vi "FringeScanner.vi"() -> ()   [LabVIEW 2009, in "FringeScanner.lvlib"]
uses:
  FringeScanner.lvlib
  Nicmos/Controls/NICMOS.READOUT.ctl
panel:
  in  "Wavelength":dbl[unit]=1.3e-06
  in  "Frame per fringe":dbl=5.0
  in  "STOP button":bool
  in  "UPDATE button":bool
  out "OPD per pixel":dbl[unit]
  out "Actual":T1
  in  "Autcollimation":bool=TRUE
  out "OPD stroke":dbl[unit]
  in  "Requested":T1={"Readout"=100, "Deglitch"=10, "Framerate"=200.0, "Bank"=2}
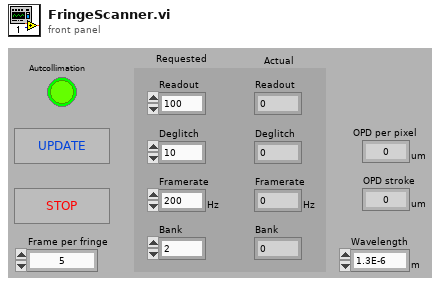
[diagram p1: front panel]
types:
  T1 = typedef "NICMOS.READOUT.ctl" = cluster{"Readout":i32, "Deglitch":i32, "Framerate":dbl[unit], "Bank":i32}
  T2 = typedef "PIEZO.WAVE.ctl" = cluster{"Speed":dbl[unit], "Stiffness (0.95)":dbl, "Linear Stroke":dbl[unit], "Delay":dbl[unit]}
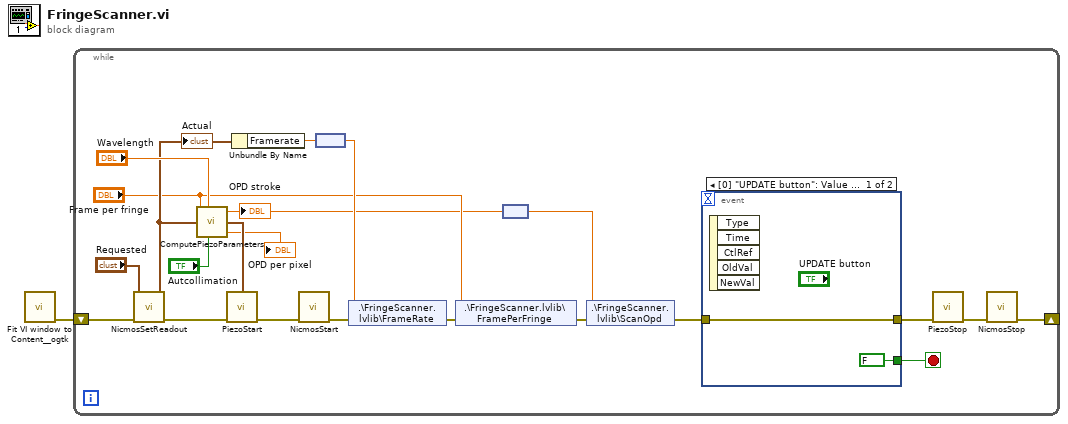
[diagram p0: block diagram]
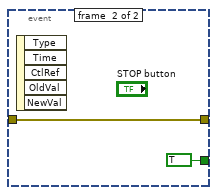
[diagram p2: hidden frame]
diagram:
  n1 = call <userlib>:"Fit VI window to Content__ogtk.vi"() -> ("error out"=w1:errorcluster)  [unwired: 6 in, 1 out]
  n2 = while {
    shift-right: [w22] -> _
    shift-left: w1 -> [w23]
    stop <- w12 stop-if-true
    n3 = call "NicmosSetReadout.vi"("READOUT in"="Requested", "error in (no error)"=w23) -> ("READOUT out"=w11:T1, "error out"=w18:errorcluster)  [unwired: 6 in]
    "Actual" <- w11
    n4 = call "ComputePiezoParameters.vi"("Frame per fringe"="Frame per fringe", "Wavelength"="Wavelength", "READOUT"=w11, "Autcollimation"="Autcollimation") -> ("OPD stroke"=w3:dbl[unit], "WAVE"=w16:T2, "OPD per pixel"=→"OPD per pixel":dbl[unit])  [unwired: 1 in]
    "OPD stroke" <- w3
    n5 = call "PiezoStart.vi"("WAVE"=w16, "error in (no error)"=w18) -> ("error out"=w17:errorcluster)  [unwired: 7 in]
    n6 = Unbundle By Name(w11) -> ("Framerate"=w10:dbl[unit])
    n7 = call "NicmosStart.vi"("error in (no error)"=w17) -> ("error out"=w9:errorcluster)  [unwired: 8 in]
    n8 = node(w10) -> (w8:dbl)
    n9 = shared-variable ".\\FringeScanner.lvlib\\FrameRate"(w8, error in=w9) -> (error out=w7:errorcluster)
    n10 = shared-variable ".\\FringeScanner.lvlib\\FramePerFringe"("Frame per fringe", error in=w7) -> (error out=w6:errorcluster)
    n11 = node(w3) -> (w2:dbl)
    n12 = shared-variable ".\\FringeScanner.lvlib\\ScanOpd"(w2, error in=w6) -> (error out=w5:errorcluster)
    n13 = event shown="[0] \"UPDATE button\": Value Change" {
      selector: _ -> [_ _]
      dyn-events: _ -> [_ _]
      timeout: _ -> [_ _]
      tunnel: w5 -> [w25 w27]
      tunnel: [w25 w27] -> w13
      tunnel: [FALSE TRUE] -> w12
      event #0 {
        n14 = event-data() -> ()  [unwired: 1 in, 5 out]
      }
      event #1 {
        n15 = event-data() -> ()  [unwired: 1 in, 5 out]
      }
    }
    n16 = call "PiezoStop.vi"("error in (no error)"=w13) -> ("error out"=w15:errorcluster)  [unwired: 10 in]
    n17 = call "NicmosStop.vi"("error in (no error)"=w15) -> ("error out"=w22:errorcluster)  [unwired: 8 in]
  }
